vi "Generate Observer.vi"(8 "error in":errorcluster, 11 "Data Subject in":refnum<class "Publisher.lvclass">) -> (0 "error out":errorcluster, 2 "Observer":refnum<queue>, 3 "Data Subject out":refnum<class "Publisher.lvclass">)   [LabVIEW 2014, in "Publisher.lvclass"]
doc: "This VI generates a queue containing a DVR of the Base Data class. The reference to the queue generated is added to the list of queues maintained by the subject class. The queue can be used by interested classes that wish to subscribe to the data monitored by the subject class."
uses:
  Publisher.lvclass
  Data/Data.lvclass
  Publisher.lvclass/Publisher.ctl
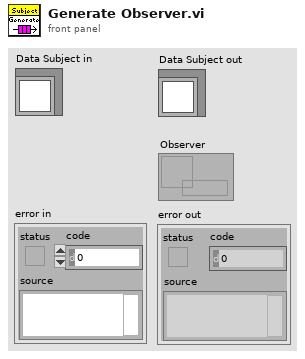
[diagram p1: front panel]
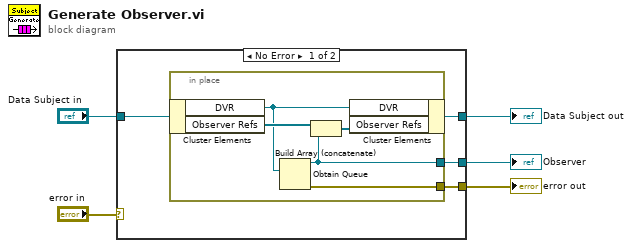
[diagram p0: block diagram]
diagram:
  n1 = case shown="No Error" "error in" {
    selector: "error in" -> [_ w16]
    tunnel: [w6 w16] -> w4
    tunnel: [w7 w15] -> w2
    tunnel: "Data Subject in" -> [w9 w15]
    tunnel: [w8 _] -> w1
    frame No Error {
      n2 = in-place {
        in-place-border: [w13] -> w8
        in-place-border: [w10] -> w6
        n3 = in-place-cluster #1(w9) -> ("DVR"=w11:refnum<data-value>, "Observer Refs"=w14:refnum<queue>[])
        n4 = Obtain Queue(element data type=w11) -> (queue out=w13:refnum<queue>, error out=w10:errorcluster)  [unwired: 4 in, 1 out]
        n5 = Build Array (concatenate)(w14, w13) -> (w12:refnum<queue>[])
        n6 = in-place-cluster #1("DVR"=w11, "Observer Refs"=w12) -> (w7:refnum<class "Publisher.lvclass">)
      }
    }
    frame Error {
    }
  }
  "error out" <- w4
  "Data Subject out" <- w2
  "Observer" <- w1
